vi "Keyboard button size.vi"(8 "error in (no error)":errorcluster) -> (0 "error out":errorcluster, 1 "Key Spacing":dbl, 2 "Key Width":dbl, 3 "Key Height":dbl)   [LabVIEW 2014]
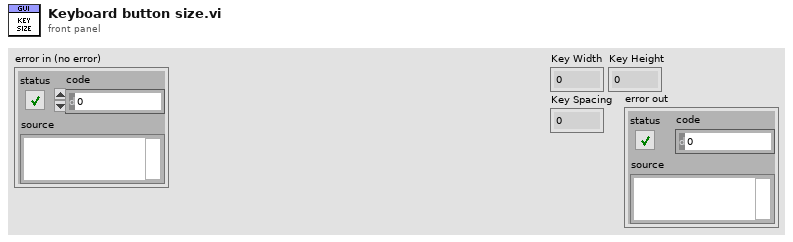
[diagram p1: front panel]
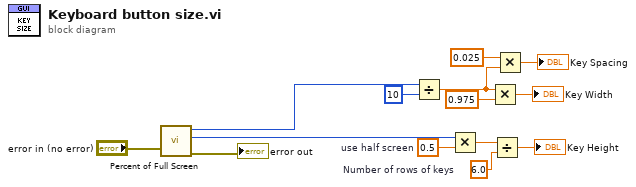
[diagram p0: block diagram]
diagram:
  w7 = 6.0  # Number of rows of keys
  w9 = 0.5  # use half screen
  n1 = call "Percent of Full Screen.vi"("error in (no error)"="error in (no error)") -> ("error out"=→"error out":errorcluster, "Bottom"=w10:i16, "Right"=w13:i16)  [unwired: 8 in]
  n2 = Divide(x=w13, y=i16 10) -> (x/y=w4:dbl)
  n3 = Multiply(x=w10, y=w9) -> (x*y=w8:dbl)
  n4 = Multiply(x=w4, y=0.975) -> (x*y=→"Key Width":dbl)
  n5 = Divide(x=w8, y=w7) -> (x/y=→"Key Height":dbl)
  n6 = Multiply(x=0.025, y=w4) -> (x*y=→"Key Spacing":dbl)
